vi "DN4_GetErrorInformation.vi"(1 "error code":i32) -> (0 "info":string)   [LabVIEW 2020]
uses:
  DAQNavi_LV.dll
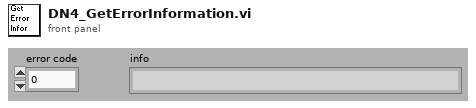
[diagram p1: front panel]
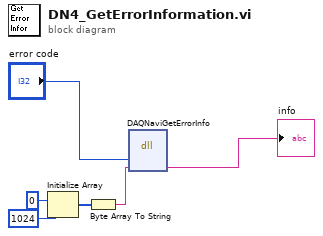
[diagram p0: block diagram]
diagram:
  n1 = Initialize Array(u8 0 ("element"), 1024 ("dimension size")) -> (w5:u8[])
  n2 = Byte Array To String(unsigned byte array=w5) -> (string=w6:string)
  n3 = dll-call lib="DAQNavi_LV.dll" fn="DAQNaviGetErrorInfo"("err"="error code", "info"=w6) -> ("info"=→"info":string)  [unwired: 4 in, 3 out]
